vi "Drying_FGV.vi"(7 "Command":enum16{"SET", "GET"}(ring), 8 "error in (no error)":errorcluster, 11 "Elapsed_Time(s)":dbl) -> (0 "error out":errorcluster, 3 "Elapsed_Time(s)_OUT":dbl)   [LabVIEW 2017]
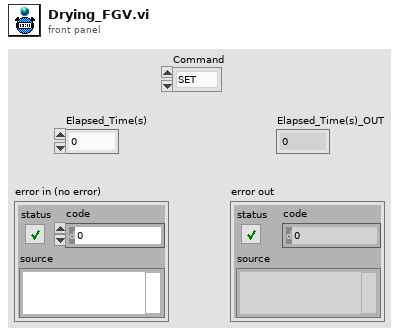
[diagram p1: front panel]
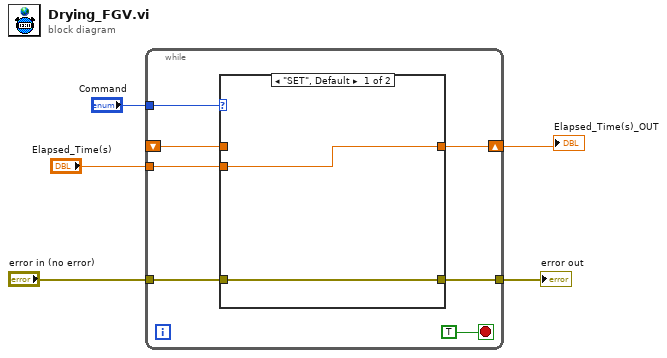
[diagram p0: block diagram]
diagram:
  n1 = while {
    tunnel: [w12] -> w5
    tunnel: "error in (no error)" -> [w11]
    shift-right: [w9] -> w2
    shift-left: _ -> [w7]
    tunnel: "Command" -> [w10]
    tunnel: "Elapsed_Time(s)" -> [w8]
    stop <- TRUE stop-if-true
    n2 = case shown="\"SET\", Default" w10 {
      tunnel: [w14 w16] -> w12
      tunnel: w11 -> [w14 w16]
      tunnel: [w13 w15] -> w9
      tunnel: w8 -> [w13 _]
      tunnel: w7 -> [_ w15]
      frame "SET", Default {
      }
      frame "GET" {
      }
    }
  }
  "Elapsed_Time(s)_OUT" <- w2
  "error out" <- w5
